vi "Generate Arduino Data.vi"(8 "error in (no error)":errorcluster, 9 "t0":timestamp, 11 "VISA resource name in":refnum<visa-resource-name>) -> (0 "error out":errorcluster, 1 "next t0":timestamp, 2 "Graph Data":waveform(dbl)[](array[waveform]), 3 "VISA resource name out":refnum<visa-resource-name>)   [LabVIEW 2017, in "Acquisition.lvlib"]
doc: "Generates sample waveforms according to the signal type in the HW Config input."
uses:
  Acquisition.lvlib
panel:
  out "read buffer":string
  out "return count":u32
  out "length":i32
  out "Waveform Chart 2":u32(graph)
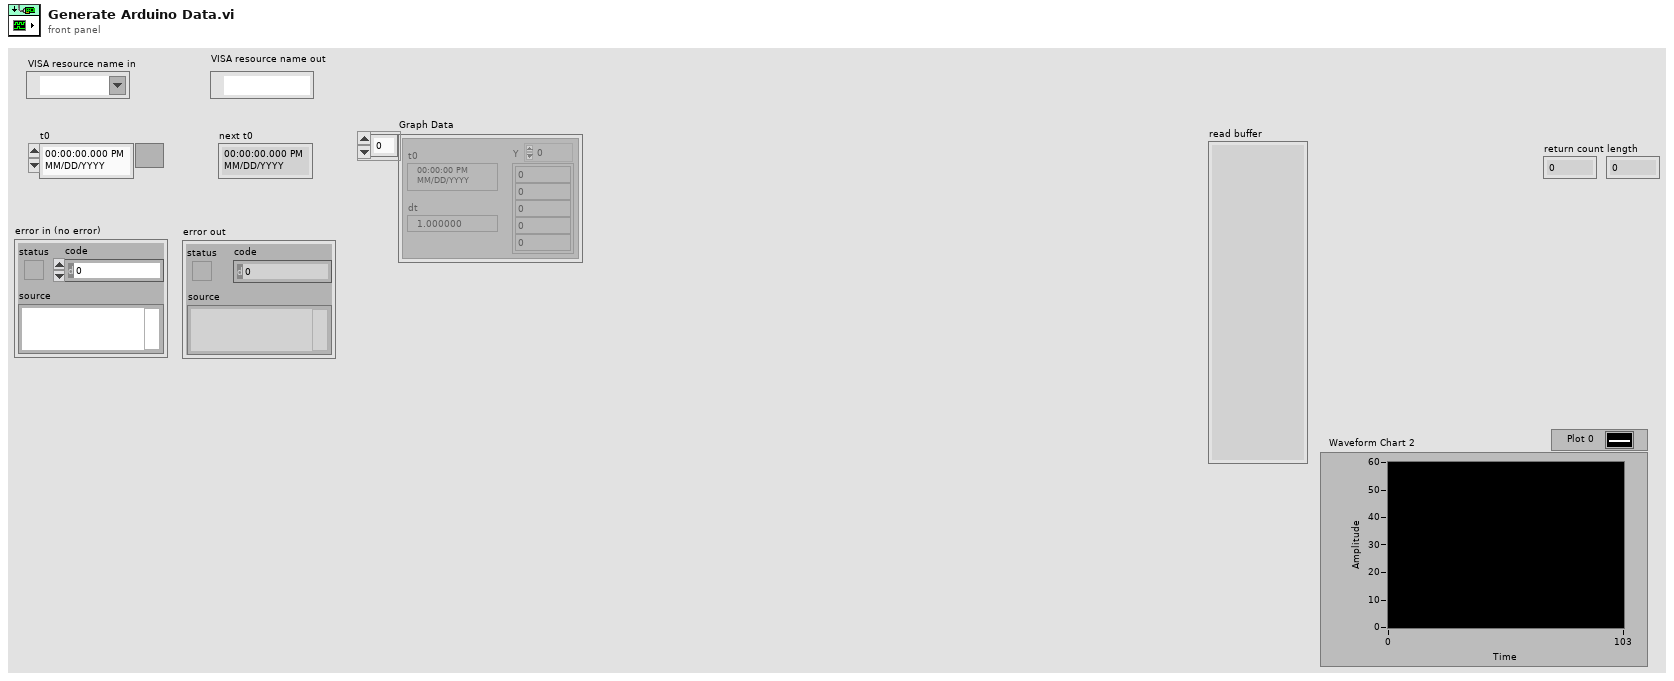
[diagram p1: front panel]
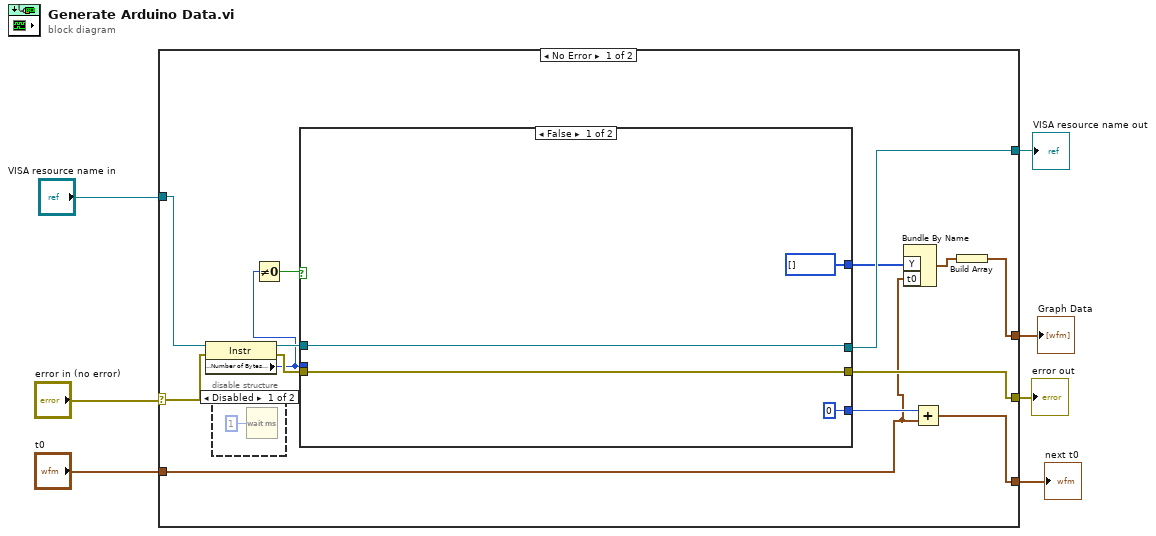
[diagram p0: block diagram]
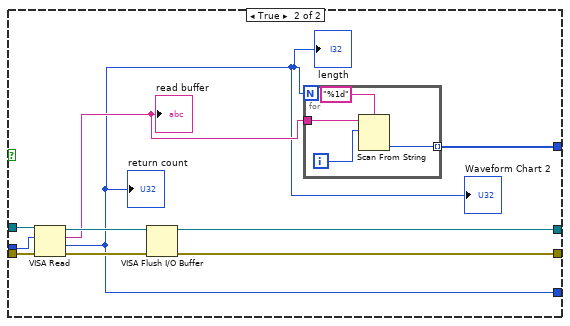
[diagram p3: hidden frame]
diagram:
  n1 = case shown="No Error" "error in (no error)" {
    selector: "error in (no error)" -> [w16 w42]
    tunnel: [w14 w42] -> w6
    tunnel: "VISA resource name in" -> [w17 w41]
    tunnel: [w15 w41] -> w4
    tunnel: [w11 _] -> w3
    tunnel: "t0" -> [w8 _]
    tunnel: [w9 _] -> w1
    frame No Error {
      n2 = property class="Instr"(reference=w17, error in=w16) -> (reference out=w21:refnum<visa-resource-name>, error out=w20:errorcluster, "Serial Settings:Number of Bytes at Serial Port"=w18:u32)
      n3 = disable-structure shown="Disabled" {
        frame Disabled {
          n4 = Wait (ms)(milliseconds to wait=u32 1) -> ()  [unwired: 1 out]
        }
        frame Enabled {
        }
      }
      n5 = Not Equal To 0?(x=w18) -> (x != 0?=w19:bool)
      n6 = case shown="False" w19 {
        tunnel: w21 -> [w26 w34]
        tunnel: w18 -> [_ w33]
        tunnel: w20 -> [w25 w32]
        tunnel: [w26 w31] -> w15
        tunnel: [w25 w30] -> w14
        tunnel: [i32[] [] w28] -> w13
        tunnel: [u32 0 ("return count") w27] -> w10
        frame False {
        }
        frame True {
          n7 = VISA Read(VISA resource name=w34, byte count=w33, error in (no error)=w32) -> (VISA resource name out=w35:refnum<visa-resource-name>, read buffer=w29:string, return count=w27:u32, error out=w36:errorcluster)
          "read buffer" <- w29
          "return count" <- w27
          "length" <- w27
          "Waveform Chart 2" <- w27
          n8 = VISA Flush I/O Buffer(VISA resource name=w35, error in (no error)=w36) -> (VISA resource name out=w31:refnum<visa-resource-name>, error out=w30:errorcluster)  [unwired: 1 in]
          n9 = for {
            N: w27 -> [_]
            tunnel: w29 -> [w40]
            tunnel: [w37] -> w28 mode=indexing
            i -> [w39]
            n10 = Scan From String(format string="%1d", input string=w40, initial scan location=w39) -> (output 1=w37:i32)  [unwired: 2 in, 3 out]
          }
        }
      }
      n11 = Bundle By Name("Y"=w13, "t0"=w8) -> (w12:waveform(i32))  [unwired: 1 in]
      n12 = Add(x=w10, y=w8) -> (x+y=w9:timestamp)
      n13 = Build Array(w12) -> (w11:waveform(i32)[])
    }
    frame Error {
    }
  }
  "error out" <- w6
  "Graph Data" <- w3
  "VISA resource name out" <- w4
  "next t0" <- w1
